vi "Read Result Data.vi"(0 "VISA resource name":refnum<visa-resource-name>, 5 "Result Number (1-200) (1)":i32=1 min=1 max=8, 11 "error in (no error)":errorcluster) -> (4 "VISA resource name out":refnum<visa-resource-name>, 6 "Test Data Cluster":T2, 15 "error out":errorcluster)   [LabVIEW 2020, in "Associated Research 78XX Series.lvlib"]
doc: "RD n? Where n is the desired step number.\n\nRetrieves the parsed data step result from the previously run test. Note you will not get a result until after the step has completed."
uses:
  <instrlib>/Associated Research 78XX Series/Associated Research 78XX Series.lvlib
  <instrlib>/Associated Research 78XX Series/Public/Configure/Steps/Low Level/ULTRA Test Type.ctl
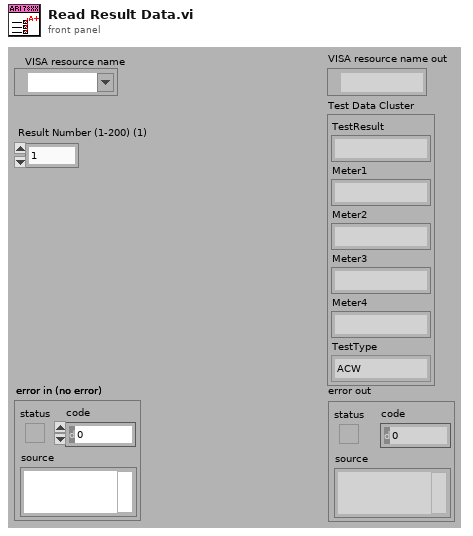
[diagram p1: front panel]
types:
  T1 = typedef "Associated Research 78XX Series.lvlib/ULTRA Test Type.ctl" = enum16{"ACW", "CONT", "DCW", "-DCW", "IR"}
  T2 = cluster{"TestResult":string, "Meter1":string, "Meter2":string, "Meter3":string, "Meter4":string, "TestType":T1}
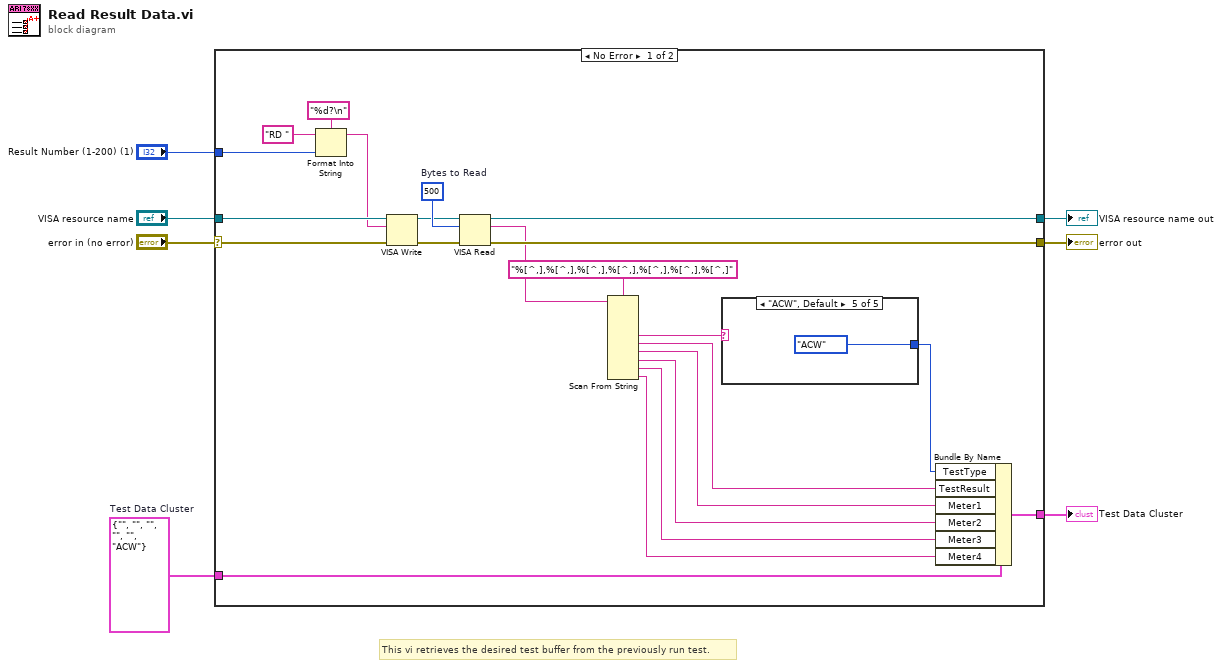
[diagram p0: block diagram]
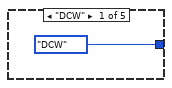
[diagram p2: hidden frame]
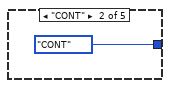
[diagram p3: hidden frame]
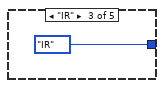
[diagram p4: hidden frame]
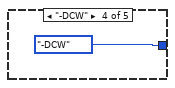
[diagram p5: hidden frame]
diagram:
  w2 = T2 {"TestResult"="", "Meter1"="", "Meter2"="", "Meter3"="", "Meter4"="", "TestType"=enum."ACW"}  # Test Data Cluster
  # "This vi retrieves the desired test buffer from the previously run test."
  n1 = case shown="No Error" "error in (no error)" {
    selector: "error in (no error)" -> [w29 w37]
    tunnel: [w26 w37] -> w6
    tunnel: [w25 w36] -> w4
    tunnel: "VISA resource name" -> [w28 w36]
    tunnel: "Result Number (1-200) (1)" -> [w27 _]
    tunnel: w2 -> [w23 w35]
    tunnel: [w22 w35] -> w1
    frame No Error {
      w18 = u32 500  # Bytes to Read
      n2 = Format Into String(format string="%d?\n", initial string="RD " ("string (\"\")"), w27) -> (resulting string=w19:string)  [unwired: 1 in, 1 out]
      n3 = VISA Write(VISA resource name=w28, write buffer=w19, error in (no error)=w29) -> (VISA resource name out=w16:refnum<visa-resource-name>, error out=w17:errorcluster)  [unwired: 1 out]
      n4 = VISA Read(VISA resource name=w16, byte count=w18, error in (no error)=w17) -> (VISA resource name out=w25:refnum<visa-resource-name>, read buffer=w24:string, error out=w26:errorcluster)  [unwired: 1 out]
      n5 = Scan From String(format string="%[^,],%[^,],%[^,],%[^,],%[^,],%[^,],%[^,]", input string=w24) -> (output 2=w9:string, output 3=w10:string, output 4=w11:string, output 5=w12:string, output 6=w13:string, output 7=w14:string)  [unwired: 10 in, 3 out]
      n6 = case shown="\"ACW\", Default" w9 {
        tunnel: [ULTRA_Test_Type."DCW" ("TestType") ULTRA_Test_Type."CONT" ("TestType") ULTRA_Test_Type."IR" ("TestType") ULTRA_Test_Type."-DCW" ("TestType") ULTRA_Test_Type."ACW" ("TestType")] -> w8
        frame "DCW" {
        }
        frame "CONT" {
        }
        frame "IR" {
        }
        frame "-DCW" {
        }
        frame "ACW", Default {
        }
      }
      n7 = Bundle By Name(cluster=w23, "TestType"=w8, "TestResult"=w10, "Meter1"=w11, "Meter2"=w12, "Meter3"=w13, "Meter4"=w14) -> (w22:T2)
    }
    frame Error {
    }
  }
  "error out" <- w6
  "VISA resource name out" <- w4
  "Test Data Cluster" <- w1
